vi "Configure Math Function.vi"   [LabVIEW 2010, in "Agilent 2000 3000 X-Series.lvlib"]
doc: "Configures the settings of math function."
uses:
  <instrlib>/Agilent 2000 3000 X-Series/Agilent 2000 3000 X-Series.lvlib
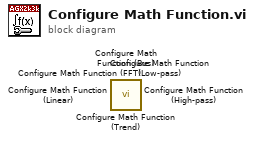
[diagram p0: block diagram]
diagram:
  n1 = call <instrlib>:"Configure Math Function (Trend).vi"() -> ()  [unwired: 10 in, 2 out]
  n2 = call <instrlib>:"Configure Math Function (Low-pass).vi"() -> ()  [unwired: 10 in, 2 out]
  n3 = call <instrlib>:"Configure Math Function (Linear).vi"() -> ()  [unwired: 10 in, 2 out]
  n4 = call <instrlib>:"Configure Math Function (High-pass).vi"() -> ()  [unwired: 10 in, 2 out]
  n5 = call <instrlib>:"Configure Math Function (FFT).vi"() -> ()  [unwired: 10 in, 2 out]
  n6 = call <instrlib>:"Configure Math Function (Bus).vi"() -> ()  [unwired: 10 in, 2 out]
